vi "Selection_SetNewData.vi"(5 "#Active Layer":i32, 6 "Fire ants event? (T)":bool=TRUE, 7 "error in":errorcluster, 8 "Highlighted?":bool, 9 "All Layers In":refnum<class "Layer.lvclass">[](array[class]), 10 "Data in":T1={"Class"={"Ants"=refnum, "Layer"=refnum, "Templates"=refnum, "Icon"=refnum, "Glyph"=refnum, "Settings"=refnum, "Tools"=refnum}, "Ref"={"Add Layer"=refnum, "Remove Layer"=refnum, "Line Text"=[], "Body Text Spec"=refnum, "DNL_Font"=refnum, "glyph path str"=refnum, "templates path str"=refnum, "Arrow Up"=refnum, "Arrow Down"=refnum, "IE VI Ref"=refnum, "Glyphs tree"=refnum, "Templates tree"=refnum, "Layer Icon Text"=refnum, "Layer Template"=refnum, "Body Text"=refnum, "Search Templates"=refnum, "TextMarker"=refnum, "Tab Control"=refnum, "Search Glyphs"=refnum, "Line Color"=refnum, "DNL_Glyphs []"=refnum, "Fill Color"=refnum, "Tools"=refnum, "Icon"=refnum, "Preview"=refnum, "Ants"=refnum, "Terminals"=refnum, "menu reference"=refnum, "LayerNames"=[], "GlyphLoadAnimation"=refnum, "TemplateLoadAnimation"=refnum, "refreshGlyphs"=refnum, "refreshTemplates"=refnum}, "Support"={"AntsRect"={"left"=0, "top"=0, "right"=0, "bottom"=0}, "Mouse Move Coords"={"Horizontal"=0, "Vertical"=0}, "Mouse Down Coords"={"Horizontal"=0, "Vertical"=0}, "Temp Coord"={"Horizontal"=0, "Vertical"=0}, "Action"=enum."Default", "Edge Color"=4914962, "Fill Color"=16860, "Mouse Down?"=FALSE, "Draft Mode?"=FALSE, "Temp Icon"=bytes[3102], "CTRL Pressed"=FALSE, "Move Selection?"=FALSE, "AntsRect Orig"={"left"=0, "top"=0, "right"=0, "bottom"=0}, "Text"="", "TM Set?"=FALSE, "Mouse inside icon?"=FALSE, "Tool (old value)"=0, "Pencil Move Color"=0, "Swap Colors?"=FALSE, "Shift pressed?"=FALSE}}) -> (0 "error out":errorcluster, 1 "User Layers":refnum<class "Layer.lvclass">[](array[class]), 3 "Data out":T1={"Class"={"Ants"=refnum, "Layer"=refnum, "Templates"=refnum, "Icon"=refnum, "Glyph"=refnum, "Settings"=refnum, "Tools"=refnum}, "Ref"={"Add Layer"=refnum, "Remove Layer"=refnum, "Line Text"=[], "Body Text Spec"=refnum, "DNL_Font"=refnum, "glyph path str"=refnum, "templates path str"=refnum, "Arrow Up"=refnum, "Arrow Down"=refnum, "IE VI Ref"=refnum, "Glyphs tree"=refnum, "Templates tree"=refnum, "Layer Icon Text"=refnum, "Layer Template"=refnum, "Body Text"=refnum, "Search Templates"=refnum, "TextMarker"=refnum, "Tab Control"=refnum, "Search Glyphs"=refnum, "Line Color"=refnum, "DNL_Glyphs []"=refnum, "Fill Color"=refnum, "Tools"=refnum, "Icon"=refnum, "Preview"=refnum, "Ants"=refnum, "Terminals"=refnum, "menu reference"=refnum, "LayerNames"=[], "GlyphLoadAnimation"=refnum, "TemplateLoadAnimation"=refnum, "refreshGlyphs"=refnum, "refreshTemplates"=refnum}, "Support"={"AntsRect"={"left"=0, "top"=0, "right"=0, "bottom"=0}, "Mouse Move Coords"={"Horizontal"=0, "Vertical"=0}, "Mouse Down Coords"={"Horizontal"=0, "Vertical"=0}, "Temp Coord"={"Horizontal"=0, "Vertical"=0}, "Action"=enum."Default", "Edge Color"=4914962, "Fill Color"=16860, "Mouse Down?"=FALSE, "Draft Mode?"=FALSE, "Temp Icon"=bytes[3102], "CTRL Pressed"=FALSE, "Move Selection?"=FALSE, "AntsRect Orig"={"left"=0, "top"=0, "right"=0, "bottom"=0}, "Text"="", "TM Set?"=FALSE, "Mouse inside icon?"=FALSE, "Tool (old value)"=0, "Pencil Move Color"=0, "Swap Colors?"=FALSE, "Shift pressed?"=FALSE}}, 4 "Remaining Indices":i32[](array[numeric]))   [LabVIEW 2021]
uses:
  <vilib>/LabVIEW Icon API/lv_icon/Classes/Layer/Layer.lvclass
  <resource>/plugins/NIIconEditor/Controls/Global Data.ctl
  <resource>/plugins/NIIconEditor/Class/Ants/Ants.lvclass
  <resource>/plugins/NIIconEditor/Class/FakedArray/FakedArray.lvclass
  <vilib>/LabVIEW Icon API/lv_icon/Classes/Icon/Icon.lvclass
  <resource>/plugins/NIIconEditor/Class/Icon Library/Glyph.lvclass
  <resource>/plugins/NIIconEditor/Class/Settings/Settings.lvclass
  <resource>/plugins/NIIconEditor/Class/Tools/Tools Paint.lvclass
  <resource>/plugins/NIIconEditor/Controls/IE Classes.ctl
  <resource>/plugins/NIIconEditor/Controls/References Cluster.ctl
  <resource>/plugins/NIIconEditor/Controls/SupportClass.ctl
  <vilib>/Utility/miscctls.llb/LVPoint32TypeDef.ctl
  <resource>/plugins/NIIconEditor/Controls/SupportClass_Action.ctl
  <vilib>/LabVIEW Icon API/lv_icon/Controls/IEColor.ctl
  <vilib>/LabVIEW Icon API/lv_icon/Classes/Icon Framework/Icon Framework.lvclass
  <vilib>/LabVIEW Icon API/lv_icon/lv_icon.lvlib
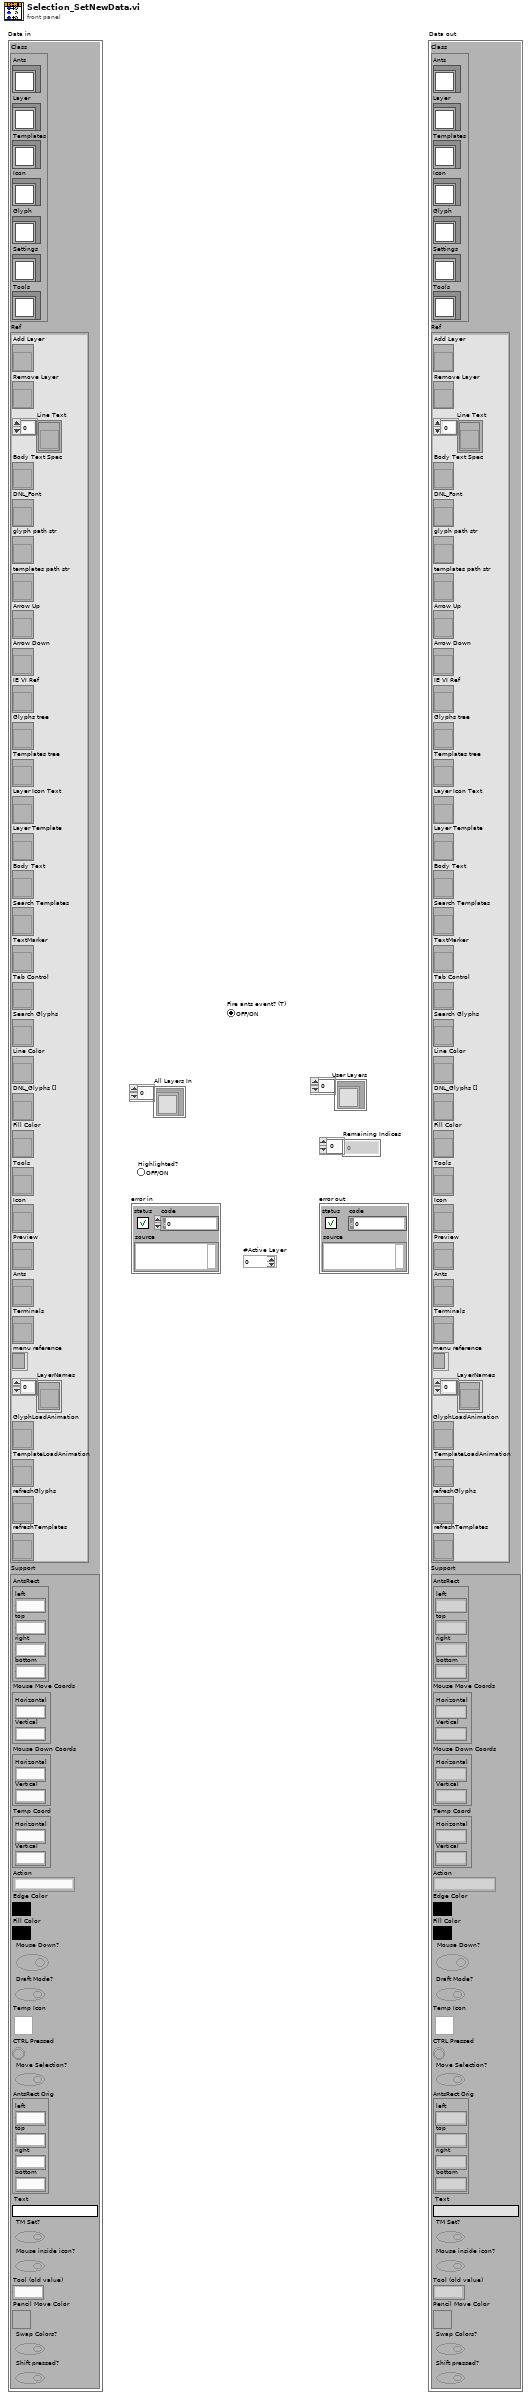
[diagram p1: front panel]
types:
  T1 = typedef "lv_icon.lvlib/Global Data.ctl" = cluster{"Class":T2, "Ref":T3, "Support":T4}
  T2 = typedef "IE Classes.ctl" = cluster{"Ants":refnum<class "Ants.lvclass">, "Layer":refnum<class "FakedArray.lvclass">, "Templates":refnum<class "FakedArray.lvclass">, "Icon":refnum<class "Icon.lvclass">, "Glyph":refnum<class "Glyph.lvclass">, "Settings":refnum<class "Settings.lvclass">, "Tools":refnum<class "Tools Paint.lvclass">}
  T3 = typedef "lv_icon.lvlib/References Cluster.ctl" = cluster{"Add Layer":refnum<vi>, "Remove Layer":refnum<vi>, "Line Text":refnum<vi>[], "Body Text Spec":refnum<vi>, "DNL_Font":refnum<vi>, "glyph path str":refnum<vi>, "templates path str":refnum<vi>, "Arrow Up":refnum<vi>, "Arrow Down":refnum<vi>, "IE VI Ref":refnum<vi>, "Glyphs tree":refnum<vi>, "Templates tree":refnum<vi>, "Layer Icon Text":refnum<vi>, "Layer Template":refnum<vi>, "Body Text":refnum<vi>, "Search Templates":refnum<vi>, "TextMarker":refnum<vi>, "Tab Control":refnum<vi>, "Search Glyphs":refnum<vi>, "Line Color":refnum<vi>, "DNL_Glyphs []":refnum<vi>, "Fill Color":refnum<vi>, "Tools":refnum<vi>, "Icon":refnum<vi>, "Preview":refnum<vi>, "Ants":refnum<vi>, "Terminals":refnum<vi>, "menu reference":refnum<k9>, "LayerNames":refnum<vi>[], "GlyphLoadAnimation":refnum<vi>, "TemplateLoadAnimation":refnum<vi>, "refreshGlyphs":refnum<vi>, "refreshTemplates":refnum<vi>}
  T4 = typedef "SupportClass.ctl" = cluster{"AntsRect":cluster{"left":i16, "top":i16, "right":i16, "bottom":i16}, "Mouse Move Coords":T5, "Mouse Down Coords":T5, "Temp Coord":T5, "Action":T6, "Edge Color":T7, "Fill Color":T7, "Mouse Down?":bool, "Draft Mode?":bool, "Temp Icon":picture, "CTRL Pressed":bool, "Move Selection?":bool, "AntsRect Orig":cluster{"left":i16, "top":i16, "right":i16, "bottom":i16}, "Text":string, "TM Set?":bool, "Mouse inside icon?":bool, "Tool (old value)":u32, "Pencil Move Color":u32, "Swap Colors?":bool, "Shift pressed?":bool}
  T5 = typedef "LVPoint32TypeDef.ctl" = cluster{"Horizontal":i32, "Vertical":i32}
  T6 = typedef "SupportClass_Action.ctl" = enum16{"Default", "Move Selection", "Glyph Library", "Tool"}
  T7 = typedef "IEColor.ctl" = u32
  T8 = typedef "Layer.ctl" = cluster{"LayerIcon":picture, "LayerName":string, "Opacity":u8, "Visibility?":bool}
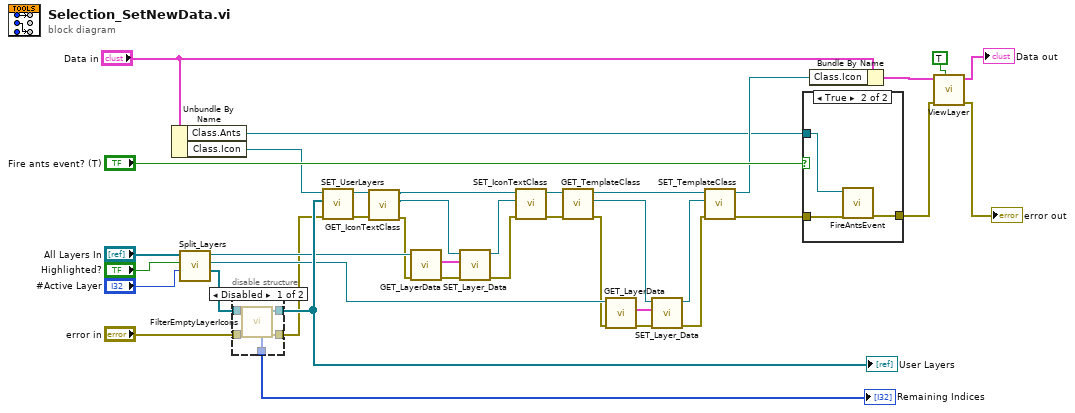
[diagram p0: block diagram]
diagram:
  n1 = Unbundle By Name("Data in") -> ("Class.Ants"=w8:refnum<class "Ants.lvclass">, "Class.Icon"=w11:refnum<class "Icon.lvclass">)
  n2 = call <resource>:"Split_Layers.vi"("#Active Layer"="#Active Layer", "Is Highlighted?"="Highlighted?", "Layer out"="All Layers In") -> ("User Layers"=w33:refnum<class "Layer.lvclass">[], "Template"=w28:refnum<class "Layer.lvclass">, "Icon Text"=w31:refnum<class "Layer.lvclass">)  [unwired: 6 out]
  n3 = disable-structure shown="Disabled" {
    disable-tunnel: w33 -> [w44 w46]
    disable-tunnel: [w43 w46] -> w32
    disable-tunnel: [w42 w45] -> w14
    disable-tunnel: [w41 _] -> w12
    disable-tunnel: "error in" -> [w40 w45]
    frame Disabled {
      n4 = call <vilib>:"FilterEmptyLayerIcons.vi"("error in (no error)"=w40, "Layers"=w44) -> ("error out"=w42:errorcluster, "Layers out"=w43:refnum<class "Layer.lvclass">[], "Remaining Indices"=w41:i32[])  [unwired: 7 out]
    }
    frame Enabled {
    }
  }
  "User Layers" <- w32
  "Remaining Indices" <- w12
  n5 = call-dynamic "SET_UserLayers.vi"("error in (no error)"=w14, "Layers"=w32, "Icon.lvclass in"=w11) -> ("error out"=w19:errorcluster, "Icon.lvclass out"=w18:refnum<class "Icon.lvclass">)  [unwired: 7 in]
  n6 = call-dynamic "GET_IconTextClass.vi"("error in (no error)"=w19, "Icon.lvclass in"=w18) -> ("error out"=w15:errorcluster, "Icon Framework.lvclass"=w16:refnum<class "Icon Framework.lvclass">, "Icon.lvclass out"=w17:refnum<class "Icon.lvclass">)  [unwired: 7 out]
  n7 = call-dynamic "GET_LayerData.vi"("error in (no error)"=w15, "Layer.lvclass in"=w31) -> ("error out"=w24:errorcluster, "Data"=w30:T8)  [unwired: 8 out]
  n8 = call-dynamic "SET_Layer_Data.vi"("error in (no error)"=w24, "Data"=w30, "Layer.lvclass in"=w16) -> ("error out"=w23:errorcluster, "Layer.lvclass out"=w29:refnum<class "Icon Framework.lvclass">)  [unwired: 1 in, 6 out]
  n9 = call-dynamic "SET_IconTextClass.vi"("error in (no error)"=w23, "Icon Framework.lvclass"=w29, "Icon.lvclass in"=w17) -> ("error out"=w35:errorcluster, "Icon.lvclass out"=w36:refnum<class "Icon.lvclass">)  [unwired: 7 out]
  n10 = call-dynamic "GET_TemplateClass.vi"("error in (no error)"=w35, "Icon.lvclass in"=w36) -> ("error out"=w22:errorcluster, "Icon Framework.lvclass"=w26:refnum<class "Icon Framework.lvclass">, "Icon.lvclass out"=w37:refnum<class "Icon.lvclass">)  [unwired: 7 out]
  n11 = call-dynamic "GET_LayerData.vi"("error in (no error)"=w22, "Layer.lvclass in"=w28) -> ("error out"=w21:errorcluster, "Data"=w27:T8)  [unwired: 8 out]
  n12 = call-dynamic "SET_Layer_Data.vi"("error in (no error)"=w21, "Data"=w27, "Layer.lvclass in"=w26) -> ("error out"=w20:errorcluster, "Layer.lvclass out"=w25:refnum<class "Icon Framework.lvclass">)  [unwired: 1 in, 6 out]
  n13 = call-dynamic "SET_TemplateClass.vi"("error in (no error)"=w20, "Icon Framework.lvclass"=w25, "Icon.lvclass in"=w37) -> ("error out"=w1:errorcluster, "Icon.lvclass out"=w9:refnum<class "Icon.lvclass">)  [unwired: 7 out]
  n14 = case shown="True" "Fire ants event? (T)" {
    tunnel: [w47 w50] -> w3
    tunnel: w1 -> [w47 w49]
    tunnel: w8 -> [_ w48]
    frame False {
    }
    frame True {
      n15 = call <resource>:"FireAntsEvent.vi"("error in (no error)"=w49, "Ants in"=w48) -> ("error out"=w50:errorcluster)  [unwired: 2 in, 7 out]
    }
  }
  n16 = Bundle By Name(cluster="Data in", "Class.Icon"=w9) -> (w5:T1)
  n17 = call <resource>:"ViewLayer.vi"("Add to Undo?"=TRUE, "error in (no error)"=w3, "Data in"=w5) -> ("error out"=→"error out":errorcluster, "Data out"=→"Data out":T1)  [unwired: 1 in, 6 out]
